vi "Proportional Control RIGHT.vi"(2 "output range":cluster{"Max":dbl, "Min":dbl}={"Max"=1.0, "Min"=-1.0}, 3 "Gain":dbl=0.2, 4 "process variable":dbl=175.6597521072808, 5 "setpoint":dbl=180.0) -> (0 "Delta":dbl=4.340247892719191, 1 "output":dbl=0.3)   [LabVIEW 2012]
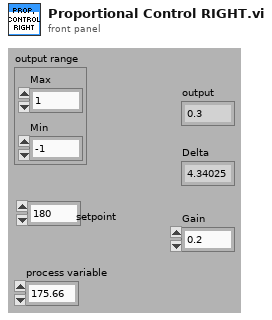
[diagram p1: front panel]
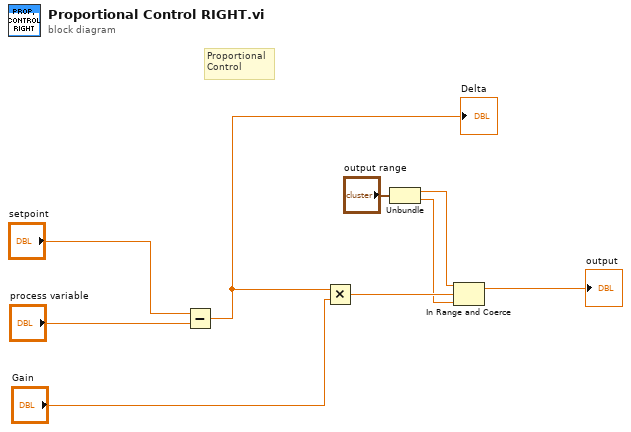
[diagram p0: block diagram]
diagram:
  # "Proportional\nControl"
  n1 = Subtract(x="setpoint", y="process variable") -> (x-y=w1:dbl)
  "Delta" <- w1
  n2 = Multiply(x=w1, y="Gain") -> (x*y=w6:dbl)
  n3 = Unbundle("output range") -> ("Max"=w4:dbl, "Min"=w3:dbl)
  n4 = In Range and Coerce(upper limit=w4, x=w6, lower limit=w3) -> (coerced(x)=→"output":dbl)  [unwired: 1 out]
